vi "BracePLUS_Serial_FileIO.vi"(5 "Serial Settings":T1={"baud rate"=115200, "data bits"=8, "parity"=enum."None", "stop bits"=10, "flow control"=0} {"flow control" items=["None"=0, "XON/XOFF"=1, "RTS/CTS"=2, "DTR/DSR"=4]; "stop bits" items=["1.0"=10, "1.5"=15, "2.0"=20]; "data bits" min=5 max=8 step=1; "baud rate" items=["75"=75, "110"=110, "134"=134, "150"=150, "300"=300, "600"=600, "1200"=1200, "1800"=1800, "2400"=2400, "4800"=4800, "7200"=7200, "9600"=9600, "14400"=14400, "19200"=19200, "28800"=28800, "38400"=38400, "56000"=56000, "57600"=57600, "115200"=115200, "128000"=128000, "230400"=230400]}, 7 "VISA resource name":refnum<visa-resource-name>="COM16", 10 "Filename to Save to...":path, 11 "Remote Filename":string) -> (0 "error out":errorcluster, 3 "Packets Recieved":i32)   [LabVIEW 2018]
panel:
  in  "Tab Control":enum32{"Display", "Debug", "Configuration"}(tab)
  out "Packets Received":i16(slide) scale=0.0..975.0
  out "Reading":bool
  out "Input Data":string
  out "read count":u32
  out "offset byte?":string
  out "Connected":bool
  out "EOF?":bool
  out "Initialised":bool
  # "ESCAPES:Upload"
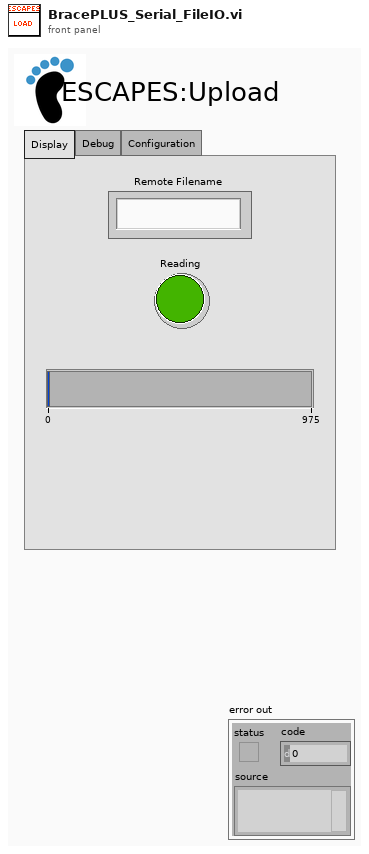
[diagram p1: front panel]
types:
  T1 = cluster{"baud rate":u32, "data bits":u16, "parity":enum16{"None", "Odd", "Even", "Mark", "Space"}, "stop bits":u16, "flow control":u16}
  T2 = enum16{"open", "replace", "create", "open or create", "replace or create", "replace or create with confirmation"}
  T3 = enum16{"big-endian, network order", "native, host order", "little-endian"}
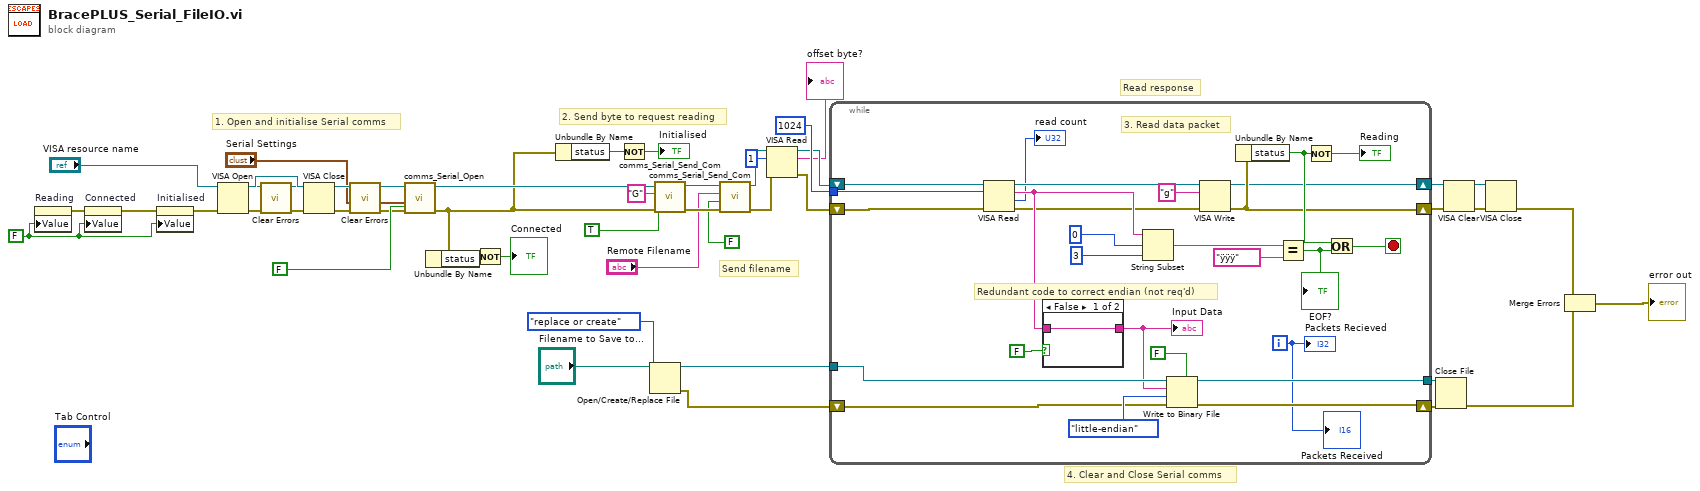
[diagram p0: block diagram]
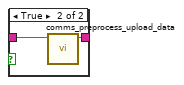
[diagram p2: hidden frame]
diagram:
  w33 = FALSE ("Send Init Comm?")
  # "Send filename"
  # "2. Send byte to request reading"
  # "Read response"
  # "4. Clear and Close Serial comms"
  # "1. Open and initialise Serial comms"
  n1 = property on="Reading" class="Bool (strict)"("Value"=w33) -> (error out=w34:errorcluster)  [unwired: 2 in, 1 out]
  n2 = property on="Connected" class="Bool (strict)"(error in=w34, "Value"=w33) -> (error out=w35:errorcluster)  [unwired: 1 in, 1 out]
  n3 = property on="Initialised" class="Bool (strict)"(error in=w35, "Value"=w33) -> (error out=w23:errorcluster)  [unwired: 1 in, 1 out]
  n4 = VISA Open(error in (no error)=w23, VISA resource name="VISA resource name") -> (VISA resource name=w32:refnum<visa-resource-name>, error out=w31:errorcluster)  [unwired: 3 in]
  n5 = call <vilib>:"Clear Errors.vi"("error in (no error)"=w31) -> ("error out"=w30:errorcluster)  [unwired: 5 in, 1 out]
  n6 = VISA Close(VISA resource name=w32, error in (no error)=w30) -> (error out=w29:errorcluster)
  n7 = call <vilib>:"Clear Errors.vi"("error in (no error)"=w29) -> ("error out"=w28:errorcluster)  [unwired: 5 in, 1 out]
  n8 = call "comms_Serial_Open.vi"("Send Init Comm?"=FALSE, "error in (no error)"=w28, "Serial Settings in"="Serial Settings", "VISA Refnum in"="VISA resource name") -> ("error out"=w17:errorcluster, "VISA Refnum out"=w18:refnum<visa-resource-name>)  [unwired: 5 in, 1 out]
  n9 = Unbundle By Name(w17) -> ("status"=w39:bool)
  n10 = Not(x=w39) -> (.not. x?=→"Connected":bool)
  n11 = Unbundle By Name(w17) -> ("status"=w38:bool)
  n12 = Not(x=w38) -> (.not. x?=→"Initialised":bool)
  n13 = Open/Create/Replace File(file path (use dialog)="Filename to Save to...", operation (0:open)=T2."replace or create") -> (refnum out=w14:refnum<file>, error out=w13:errorcluster)  [unwired: 4 in, 1 out]
  n14 = call "comms_Serial_Send_Com.vi"("error in"=w17, "Buffer Clear?"=TRUE, "Command"="G", "VISA resource in"=w18) -> ("error out"=w22:errorcluster, "VISA resource Out"=w20:refnum<visa-resource-name>)  [unwired: 5 in, 1 out]
  n15 = call "comms_Serial_Send_Com.vi"("error in"=w22, "Buffer Clear?"=FALSE, "Command"="Remote Filename", "VISA resource in"=w20) -> ("error out"=w2:errorcluster, "VISA resource Out"=w9:refnum<visa-resource-name>)  [unwired: 5 in, 1 out]
  n16 = VISA Read(VISA resource name=w9, byte count=u32 1, error in (no error)=w2) -> (VISA resource name out=w8:refnum<visa-resource-name>, read buffer=→"offset byte?":string, error out=w3:errorcluster)  [unwired: 1 out]
  n17 = while {
    shift-right: [w61] -> w41
    shift-left: w8 -> [w59]
    shift-right: [w63] -> w40
    shift-left: w3 -> [w58]
    tunnel: u32 1024 ("byte count") -> [w66]
    tunnel: w14 -> [w56]
    shift-right: [w55] -> w12
    shift-left: w13 -> [w48]
    tunnel: [w53] -> w11
    i -> [w45]
    stop <- w68 stop-if-true
    # "Redundant code to correct endian (not req'd)"
    # "3. Read data packet"
    n18 = VISA Read(VISA resource name=w59, byte count=w66, error in (no error)=w58) -> (VISA resource name out=w62:refnum<visa-resource-name>, read buffer=w51:string, return count=→"read count":u32, error out=w47:errorcluster)
    n19 = case shown="False" FALSE {
      tunnel: w51 -> [w72 w74]
      tunnel: [w72 w73] -> w50
      frame False {
      }
      frame True {
        n20 = call "comms_preprocess_upload_data.vi"("Binary Input Data"=w74) -> ("Binary Output (string)"=w73:string)  [unwired: 10 in]
      }
    }
    "Input Data" <- w50
    n21 = String Subset(string=w51, offset (0)=0, length (rest)=3 ("length (rest)")) -> (substring=w64:string)
    n22 = Write to Binary File(file (use dialog)=w56, data=w50, error in=w48, 5:FALSE ("prepend array or string size? (T)"), 9:T3."little-endian" ("byte order (0:big-endian, network order)")) -> (refnum out=w53:refnum<file>, error out=w55:errorcluster)  [unwired: 1 in, 1 out]
    n23 = VISA Write(VISA resource name=w62, write buffer="g", error in (no error)=w47) -> (VISA resource name out=w61:refnum<visa-resource-name>, error out=w63:errorcluster)  [unwired: 1 out]
    n24 = Unbundle By Name(w63) -> ("status"=w67:bool)
    n25 = Equal?(x=w64, y="ÿÿÿ") -> (x = y?=w69:bool)
    "EOF?" <- w69
    n26 = Not(x=w67) -> (.not. x?=→"Reading":bool)
    n27 = Or(x=w67, y=w69) -> (x .or. y?=w68:bool)
    "Packets Recieved" <- w45
    "Packets Received" <- w45
  }
  n28 = Close File(refnum=w11, error in=w12) -> (error out=w4:errorcluster)  [unwired: 1 out]
  n29 = VISA Clear(VISA resource name=w41, error in (no error)=w40) -> (VISA resource name out=w43:refnum<visa-resource-name>, error out=w42:errorcluster)
  n30 = VISA Close(VISA resource name=w43, error in (no error)=w42) -> (error out=w5:errorcluster)
  n31 = Merge Errors(w5, w4) -> (→"error out":errorcluster)
